vi "Chat Message Callback.vi"(7 "Owner":refnum<class>, 11 "Message":refnum<class "Message.lvclass">) -> (0 "error out":errorcluster)   [LabVIEW 2020, in "LV Chat Client.lvclass"]
uses:
  LV Chat Client.lvclass
  Stream-Simple-Msg/Message/Message.lvclass
  Data Types/Message.ctl
  3bb6c120-6c39-4e60-a368-f8a06dca41d0.vi
  Stream-Simple-Msg/Message/Get Data.vi
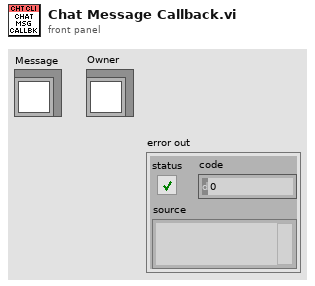
[diagram p1: front panel]
types:
  T1 = typedef "Message.ctl" = cluster{"From":string, "Time":dbl, "Message":string}
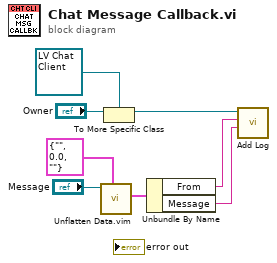
[diagram p0: block diagram]
diagram:
  n1 = call "Unflatten Data.vim"("Data Type"=T1 {"From"="", "Time"=0.0, "Message"=""} ("Message"), "Message in"="Message") -> ("Unflattened Data"=w6:T1)  [unwired: 7 in, 2 out]
  n2 = To More Specific Class(target class=refnum<class "LV Chat Client.lvclass"> refnum ("LV Chat Client.lvclass"), reference="Owner") -> (specific class reference=w3:refnum<class "LV Chat Client.lvclass">)  [unwired: 1 in, 1 out]
  n3 = Unbundle By Name(w6) -> ("From"=w2:string, "Message"=w1:string)
  n4 = call "Add Log.vi"("Message"=w1, "From (Client)"=w2, "LV Chat Client in"=w3) -> ()  [unwired: 7 in, 2 out]
